vi "lvssh2_session_callback_register_receive_64.vi"(11 "receive":refnum<vi>) -> (0 "error out":errorcluster, 2 "stop event":refnum<user-event>, 3 "user event":refnum<user-event>)   [LabVIEW 2017, in "libssh2.lvlib"]
uses:
  libssh2.lvlib
  lvssh2_session_callback_receive_function_input_args_64.ctl
  lvssh2_session_callback_receive_handler_64.vi
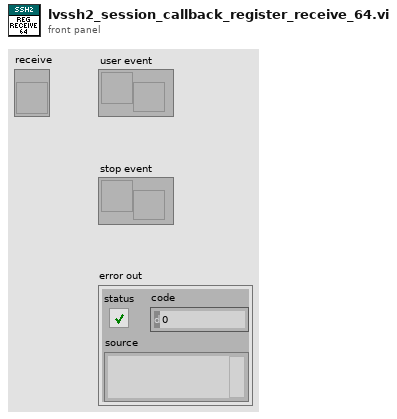
[diagram p1: front panel]
types:
  T1 = typedef "libssh2.lvlib/lvssh2_session_callback_receive_function_input_args_64.ctl" = cluster{"*socket":u64, "*buffer":u64, "length":u64, "flags":i32, "<padding>":i32, "*bytes_received":u64, "completion":u64}
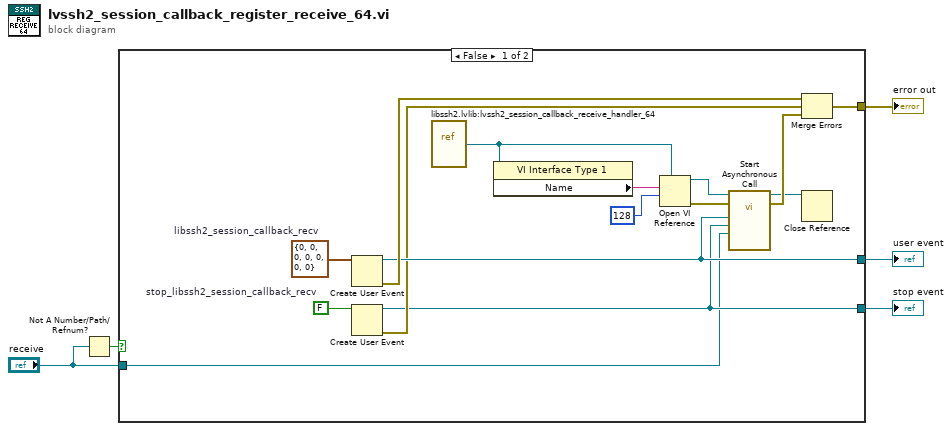
[diagram p0: block diagram]
diagram:
  n1 = Not A Number/Path/Refnum?(number/path/refnum="receive") -> (NaN/Path/Refnum?=w3:bool)
  n2 = case shown="False" w3 {
    tunnel: [w11 _] -> w5
    tunnel: [w20 _] -> w4
    tunnel: "receive" -> [w7 _]
    tunnel: [w8 _] -> w1
    frame False {
      w17 = FALSE  # stop_libssh2_session_callback_recv
      w19 = T1 {"*socket"=0, "*buffer"=0, "length"=0, "flags"=0, "<padding>"=0, "*bytes_received"=0, "completion"=0}  # libssh2_session_callback_recv
      n3 = Create User Event(user event datatype=w19) -> (user event=w11:refnum<user-event>, error out=w18:errorcluster)  [unwired: 1 in]
      n4 = Create User Event(user event datatype=w17) -> (user event=w8:refnum<user-event>, error out=w10:errorcluster)  [unwired: 1 in]
      n5 = vi-ref "libssh2.lvlib:lvssh2_session_callback_receive_handler_64.vi"() -> ("vi reference"=w12:refnum<vi>)
      n6 = property class="VI Interface Type 1"(reference=w12) -> ("Name"=w16:string)  [unwired: 1 in, 2 out]
      n7 = Open VI Reference(type specifier VI Refnum (for type only)=w12, vi path=w16, options=128) -> (vi reference=w14:refnum<vi>, error out=w15:errorcluster)  [unwired: 3 in]
      n8 = call-by-ref "Start Asynchronous Call"(reference=w14, error in=w15, "lvssh2_session_callback_receive"=w7, "Stop Event Ref"=w8, "User Event Ref"=w11) -> (reference out=w6:refnum<vi>, error out=w9:errorcluster)  [unwired: 9 in]
      n9 = Merge Errors(w18, w10, w9) -> (w20:errorcluster)
      n10 = Close Reference(reference=w6) -> ()  [unwired: 1 in, 1 out]
    }
    frame True {
    }
  }
  "user event" <- w5
  "error out" <- w4
  "stop event" <- w1
